vi "3_3_Fourier Transform of Periodic Gate.vi"() -> ()   [LabVIEW 2009]
uses:
  <vilib>/Analysis/2dsp.llb/Real FFT.vi
  <vilib>/Analysis/NI_AALPro.lvlib
panel:
  out "?":string="If the function is not periodic, then the Fourier transform will be continuous function of frequency, i.e. , x(t) is represented by the summation of all frequencies....................................................................... The fourier transform of the PULSE indicates that one sinusoid frequency  becomes indistinguishable from the next and, as a result, all frequencies must be considered."
  in  "stop":bool
  out "Magnitude spectrum":cluster{dbl, "fundamental frequency":dbl, dbl[]}(graph)={-0.0, "fundamental frequency"=0.0, [0.0, 0.0, 0.0, 0.0, 0.0, 0.0, 0.0, 0.0, 0.0, 0.0, 0.0, 0.0, 0.0, 0.0, 0.0, 0.0, 0.0, 0.0, 0.0, 0.12360679774997899, 0.0, 0.0, 0.0, 0.0, 0.0, 0.0, 0.0, 0.0, 0.0, 0.0, 0.0, 0.0, 0.0, 0.0, 0.0, 0.0, 0.0, 0.0, 0.0, 0.32360679774997897, 0.0, 0.0, 0.0, 0.0, 0.0, 0.0, 0.0, 0.0, 0.0, 0.5, 0.0, 0.0, 0.0, 0.0, 0.0, 0.0, 0.0, 0.0, 0.0, 0.32360679774997897, 0.0, 0.0, 0.0, 0.0, 0.0, 0.0, 0.0, 0.0, 0.0, 0.0, 0.0, 0.0, 0.0, 0.0, 0.0, 0.0, 0.0, 0.0, 0.0, 0.12360679774997899, 0.0, 0.0, 0.0, 0.0, 0.0, 0.0, 0.0, 0.0, 0.0, 0.0, 0.0, 0.0, 0.0, 0.0, 0.0, 0.0, 0.0, 0.0, 0.0, 0.1]}
  out "Periodic gate":dbl[](graph)=[1.0, 1.0, 1.0, 1.0, 1.0, 0.0, 0.0, 0.0, 0.0, 0.0, 1.0, 1.0, 1.0, 1.0, 1.0, 0.0, 0.0, 0.0, 0.0, 0.0, 1.0, 1.0, 1.0, 1.0, 1.0, 0.0, 0.0, 0.0, 0.0, 0.0, 1.0, 1.0, 1.0, 1.0, 1.0, 0.0, 0.0, 0.0, 0.0, 0.0, 1.0, 1.0, 1.0, 1.0, 1.0, 0.0, 0.0, 0.0, 0.0, 0.0, 1.0, 1.0, 1.0, 1.0, 1.0, 0.0, 0.0, 0.0, 0.0, 0.0, 1.0, 1.0, 1.0, 1.0, 1.0, 0.0, 0.0, 0.0, 0.0, 0.0, 1.0, 1.0, 1.0, 1.0, 1.0, 0.0, 0.0, 0.0, 0.0, 0.0, 1.0, 1.0, 1.0, 1.0, 1.0, 0.0, 0.0, 0.0, 0.0, 0.0, 1.0, 1.0, 1.0, 1.0, 1.0, 0.0, 0.0, 0.0, 0.0, 0.0]
  in  "# of samples":dbl=100.0
  in  "Time period (T)":dbl=10.0
  in  "width":dbl=5.0
  in  "Amplitude":dbl=1.0
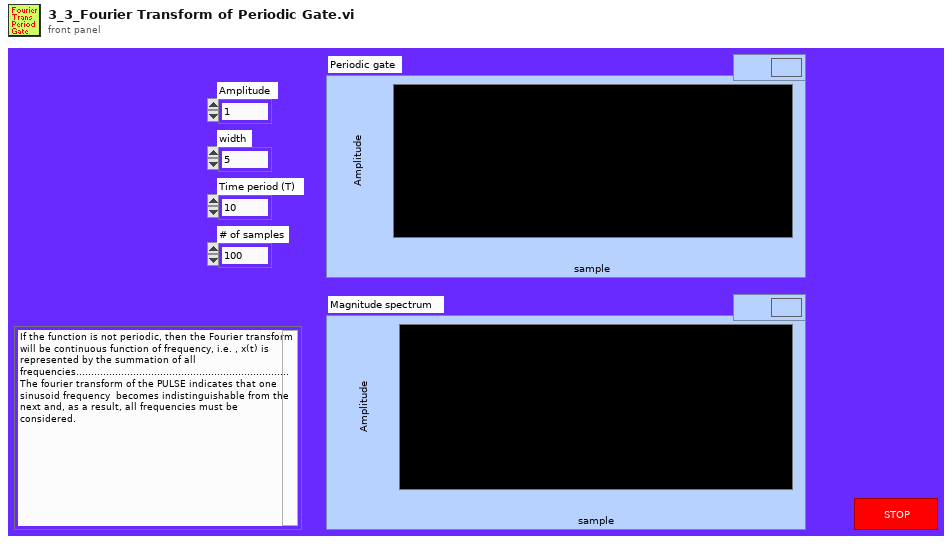
[diagram p1: front panel]
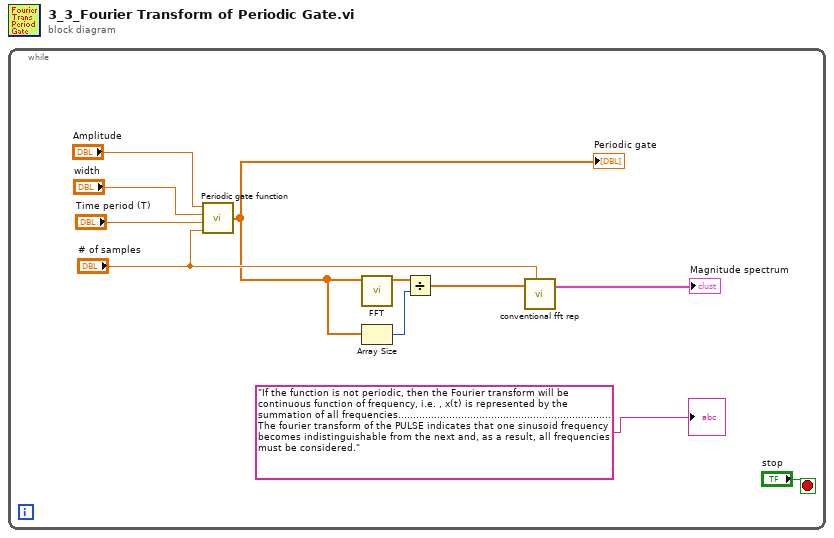
[diagram p0: block diagram]
diagram:
  n1 = while {
    stop <- "stop" stop-if-true
    n2 = call "Periodic gate function.vi"("# of samples"="# of samples", "Time period (T)"="Time period (T)", "width"="width", "Amplitude"="Amplitude") -> ("Pulse gate"=w1:dbl[])
    "Periodic gate" <- w1
    n3 = call-poly <vilib>:"FFT.vi"("X"=w1) -> ("FFT {X}"=w7:cdb[])  [unwired: 9 in, 1 out]
    n4 = Array Size(array=w1) -> (size(s)=w3:i32)
    n5 = Divide(x=w7, y=w3) -> (x/y=w4:cdb[])
    n6 = call "conventional fft rep.vi"("samples"="# of samples", "fft output"=w4) -> ("Conventional FFT mag"=→"Magnitude spectrum":cluster{dbl, "fundamental frequency":dbl, dbl[]})  [unwired: 4 in, 1 out]
    "?" <- "If the function is not periodic, then the Fourier transform will be continuous function of frequency, i.e. , x(t) is represented by the summation of all frequencies....................................................................... The fourier transform of the PULSE indicates that one sinusoid frequency  becomes indistinguishable from the next and, as a result, all frequencies must be considered."
  }
